vi "数据查询_数据查询.vi"() -> ()   [LabVIEW 2016]
uses:
  <vilib>/Utility/miscctls.llb/LVPointTypeDef.ctl
  <vilib>/Utility/miscctls.llb/LVRowAndColumnUnsignedTypeDef.ctl
  <vilib>/addons/database/_DB Variant To Data/Database Variant To Data.xnode
panel:
  in  "工作模式":string(combo)="全部数据"
  out "连接的字符串":string
  out "选中数据表":string
  in  "查询":bool
  in  "结束日期":string="2020/01/01"
  in  "起始日期":string="2010/01/01"
  out "XY图":cluster{"data":timestamp[], "data":dbl[]}[](graph)
  in  "组合框":string(combo)
  out "数据表":string[][](table)
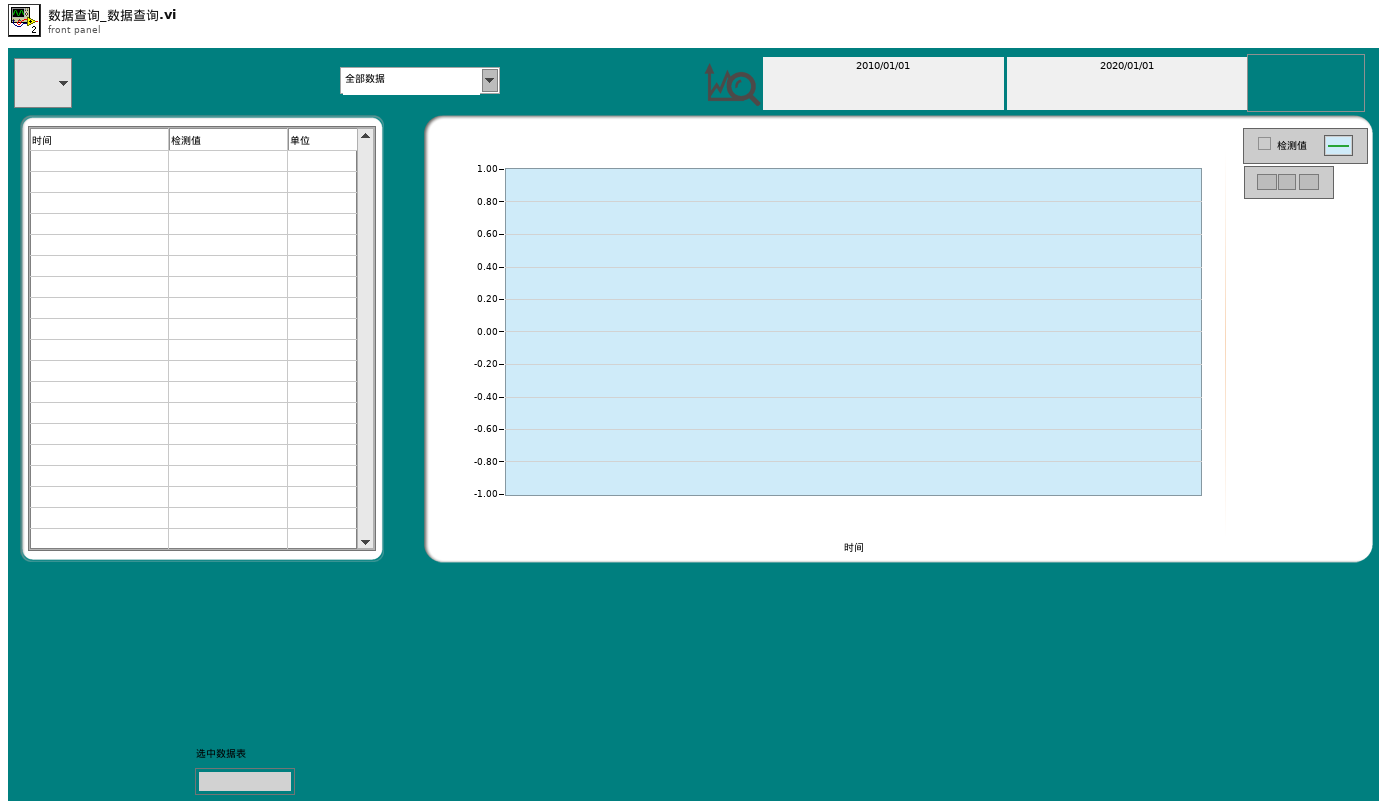
[diagram p1: front panel]
types:
  T1 = typedef "LVPointTypeDef.ctl" = cluster{"Horizontal":i16, "Vertical":i16}
  T2 = typedef "LVRowAndColumnUnsignedTypeDef.ctl" = cluster{"Row":u32, "Column":u32}
  T3 = typedef "LVPoint32TypeDef.ctl" = cluster{"Horizontal":i32, "Vertical":i32}
  T4 = typedef "LVPointDoubleTypeDef.ctl" = cluster{"Cursor X":dbl, "Cursor Y":dbl}
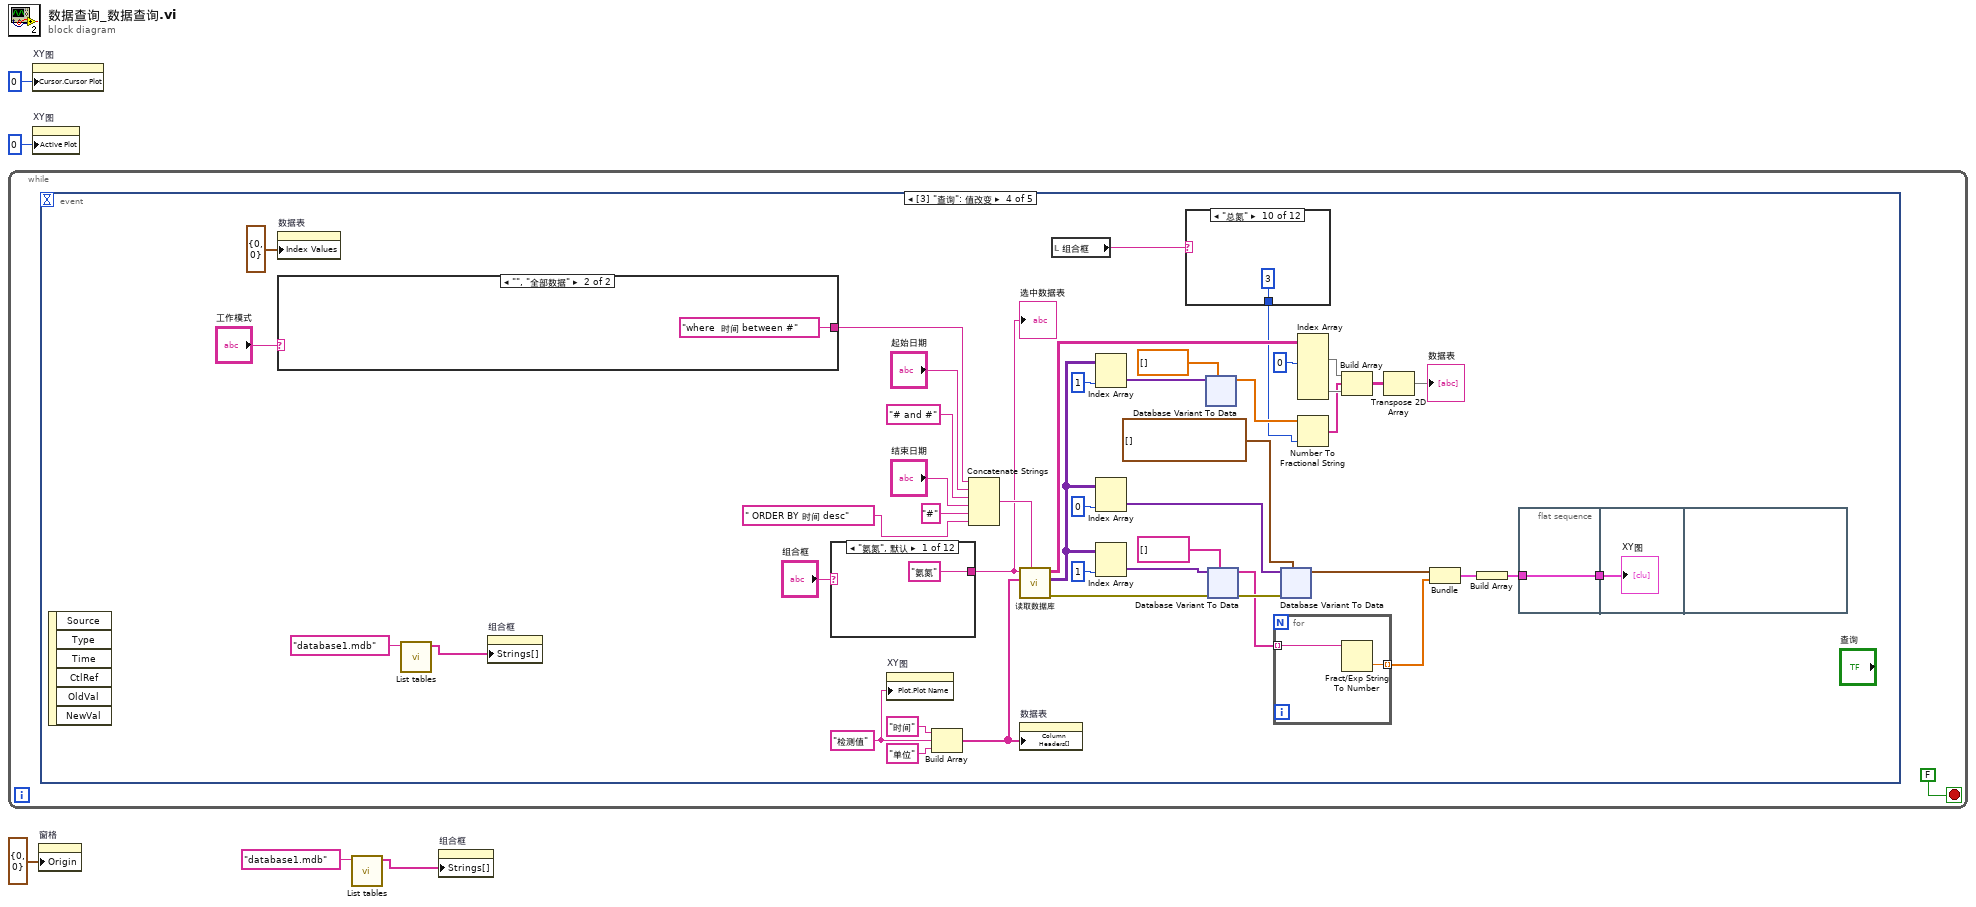
[diagram p0: block diagram]
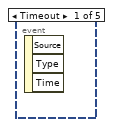
[diagram p2: hidden frame]
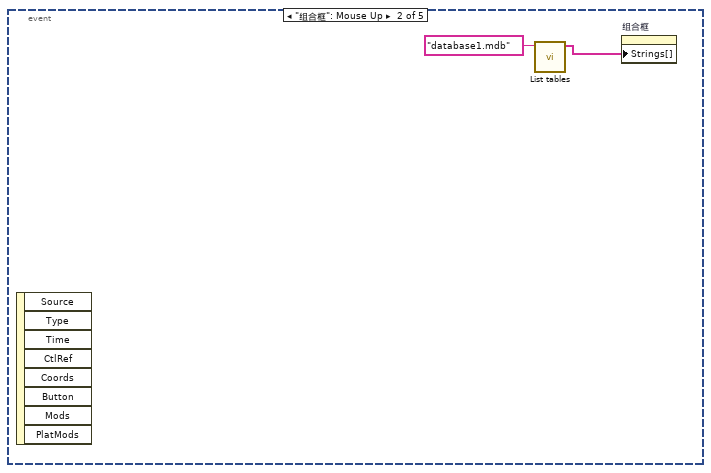
[diagram p3: hidden frame]
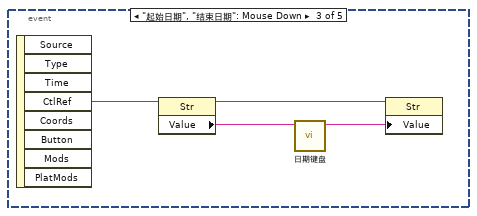
[diagram p4: hidden frame]
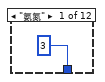
[diagram p5: hidden frame]
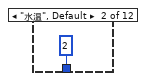
[diagram p6: hidden frame]
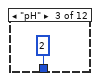
[diagram p7: hidden frame]
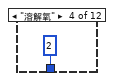
[diagram p8: hidden frame]
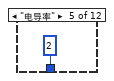
[diagram p9: hidden frame]
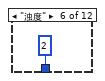
[diagram p10: hidden frame]
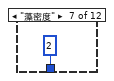
[diagram p11: hidden frame]
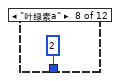
[diagram p12: hidden frame]
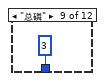
[diagram p13: hidden frame]
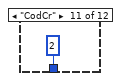
[diagram p14: hidden frame]
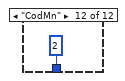
[diagram p15: hidden frame]
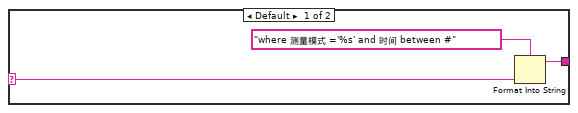
[diagram p16: hidden frame]
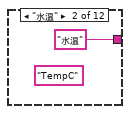
[diagram p17: hidden frame]
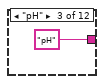
[diagram p18: hidden frame]
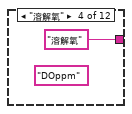
[diagram p19: hidden frame]
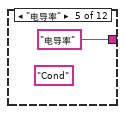
[diagram p20: hidden frame]
diagram:
  n1 = while {
    stop <- FALSE stop-if-true
    n2 = event shown="[3] \"查询\": 值改变" {
      selector: _ -> [_ _ _ _ _]
      dyn-events: _ -> [_ _ _ _ _]
      timeout: _ -> [_ _ _ _ _]
      event Timeout {
        n3 = event-data() -> ()  [unwired: 1 in, 3 out]
      }
      event "组合框": Mouse Up {
        n4 = event-data() -> ()  [unwired: 1 in, 8 out]
        n5 = call "List tables.vi"("database"="database1.mdb") -> ("tables"=w8:string[])  [unwired: 9 in, 1 out]
        n6 = property on="组合框" class="CmbBox"("Strings[]"=w8) -> ()  [unwired: 2 in, 2 out]
      }
      event "起始日期", "结束日期": Mouse Down {
        n7 = event-data() -> ("CtlRef"=w12:refnum<vi>)  [unwired: 1 in, 7 out]
        n8 = property class="Str"(reference=w12) -> (reference out=w10:refnum<vi>, "Value"=w11:string)  [unwired: 1 in, 1 out]
        n9 = call "日期键盘.vi"("原值"=w11) -> ("x+y"=w9:string)  [unwired: 10 in]
        n10 = property class="Str"(reference=w10, "Value"=w9) -> ()  [unwired: 1 in, 2 out]
      }
      event "查询": Value Change {
        w29 = "检测值"
        n11 = event-data() -> ()  [unwired: 1 in, 6 out]
        n12 = property on="数据表" class="Tbl (严格)"("Index Values"=T2 {"Row"=0, "Column"=0} ("索引值")) -> ()  [unwired: 2 in, 2 out]
        n13 = case shown="\"\", \"全部数据\"" "工作模式" {
          selector: "工作模式" -> [w72 _]
          tunnel: [w70 "where  时间 between #" ("condition")] -> w18
          frame Default {
            n14 = Format Into String(format string="where 测量模式 ='%s' and 时间 between #" ("condition"), w72) -> (resulting string=w70:string)  [unwired: 2 in, 1 out]
          }
          frame "", "全部数据" {
          }
        }
        n15 = call "List tables.vi"("database"="database1.mdb") -> ("tables"=w14:string[])  [unwired: 9 in, 1 out]
        n16 = property on="组合框" class="CmbBox"("Strings[]"=w14) -> ()  [unwired: 2 in, 2 out]
        n17 = case shown="\"氨氮\", 默认" "组合框" {
          tunnel: ["氨氮" "水温" "pH" "溶解氧" "电导率" "浊度" "藻密度" "叶绿素a" "总磷" "总氮" "CodCr" "CodMn"] -> w31
          frame "氨氮", Default {
          }
          frame "水温" {
            (unwired) "TempC"
          }
          frame "pH" {
          }
          frame "溶解氧" {
            (unwired) "DOppm"
          }
          frame "电导率" {
            (unwired) "Cond"
          }
          frame "浊度" {
            (unwired) "Turb"
          }
          frame "藻密度" {
            (unwired) "Algal"
          }
          frame "叶绿素a" {
            (unwired) "Chlor"
          }
          frame "总磷" {
            (unwired) "测量值"
          }
          frame "总氮" {
            (unwired) "测量值"
          }
          frame "CodCr" {
          }
          frame "CodMn" {
          }
        }
        "选中数据表" <- w31
        n18 = property on="XY图" class="XYGraph (严格)"("Plot.Plot Name"=w29) -> ()  [unwired: 2 in, 2 out]
        n19 = Build Array("时间", w29, "单位" ("元素")) -> (w32:string[])
        n20 = Concatenate Strings(w18, "起始日期", "# and #" ("condition"), "结束日期", "#" ("condition"), " ORDER BY 时间 desc" ("字符串")) -> (w56:string)
        n21 = call "读取数据库.vi"("condition"=w56, "显示项"=w32, "组合框"=w31) -> ("error out"=w47:errorcluster, "data"=w26:variant[][], "表格"=w39:string[][])  [unwired: 5 in, 1 out]
        n22 = property on="数据表" class="Tbl (严格)"("Column Headers[]"=w32) -> ()  [unwired: 2 in, 2 out]
        n23 = local read "组合框"() -> (w16:string)
        n24 = Index Array(array=w26, index (col)=1 ("禁用的索引 (列)")) -> (element=w24:variant[])  [unwired: 1 in]
        n25 = Index Array(array=w26, index (col)=0 ("禁用的索引 (列)")) -> (element=w50:variant[])  [unwired: 1 in]
        n26 = Index Array(array=w26, index (col)=1 ("禁用的索引 (列)")) -> (element=w48:variant[])  [unwired: 1 in]
        n27 = case shown="\"总氮\"" w16 {
          tunnel: [i16 3 ("精度(6)") i16 2 ("精度(6)") i16 2 ("精度(6)") i16 2 ("精度(6)") i16 2 ("精度(6)") i16 2 ("精度(6)") i16 2 ("精度(6)") i16 2 ("精度(6)") i16 3 ("精度(6)") i16 3 ("精度(6)") i16 2 ("精度(6)") i16 2 ("精度(6)")] -> w15
          frame "氨氮" {
          }
          frame "水温", Default {
          }
          frame "pH" {
          }
          frame "溶解氧" {
          }
          frame "电导率" {
          }
          frame "浊度" {
          }
          frame "藻密度" {
          }
          frame "叶绿素a" {
          }
          frame "总磷" {
          }
          frame "总氮" {
          }
          frame "CodCr" {
          }
          frame "CodMn" {
          }
        }
        n28 = xnode "Database Variant To Data"("database variant"=w24, "type"=sgl[] []) -> ("data"=w22:sgl[])  [unwired: 1 in, 1 out]
        n29 = xnode "Database Variant To Data"("database variant"=w48, "error in (no error)"=w47, "type"=string[] []) -> ("data"=w30:string[], "error out"=w46:errorcluster)
        n30 = for {
          tunnel: w30 -> [w113] mode=indexing
          tunnel: [w112] -> w17 mode=indexing
          n31 = Fract/Exp String To Number(string=w113) -> (number=w112:dbl)  [unwired: 3 in, 1 out]
        }
        n32 = xnode "Database Variant To Data"("database variant"=w50, "error in (no error)"=w46, "type"=timestamp[] []) -> ("data"=w41:timestamp[])  [unwired: 1 out]
        n33 = Index Array(array=w39, index (col) #1=0 ("禁用的索引 (列)")) -> (element #1=w37:string[], element #3=w27:string[])  [unwired: 5 in, 1 out]
        n34 = Number To Fractional String(number=w22, precision (6)=w15) -> (F-format string=w21:string[])  [unwired: 2 in]
        n35 = Build Array(w37, w21, w27) -> (w36:string[][])
        n36 = Transpose 2D Array(2D array=w36) -> (transposed array=→"数据表":string[][])
        n37 = Bundle("data"=w41, w17) -> (w42:cluster{"data":timestamp[], dbl[]})  [unwired: 1 in]
        n38 = Build Array(w42) -> (w43:cluster{"data":timestamp[], dbl[]}[])
        n39 = flat-sequence {
          tunnel: [w126] -> w44
          tunnel: w43 -> [w126]
          tunnel: w44 -> [w127]
          frame #0 {
          }
          frame #1 {
            "XY图" <- w127
          }
          frame #2 {
          }
        }
      }
      event "XY图": Mouse Move {
        w221 = "   " ("字符串")
        n40 = event-data() -> ("CtlRef"=w231:refnum<vi>, "Coords"=w230:T3)  [unwired: 1 in, 3 out]
        n41 = invoke class="XYGraph (严格)" method="Map Coords To XY"(reference=w231, "Coords"=w230) -> (reference out=w229:refnum<vi>, error out=w226:errorcluster, "XY"=w228:cluster{"X":dbl, "Y":dbl})  [unwired: 5 in, 4 out]
        n42 = property class="XYGraph (严格)"(reference=w229, error in=w226, "Cursor.Cursor Position"=w228) -> (error out=w227:errorcluster)  [unwired: 1 out]
        n43 = property on="XY图" class="XYGraph (严格)"(error in=w227) -> ("Cursor.Cursor Position"=w224:T4)  [unwired: 1 in, 2 out]
        n44 = Unbundle(w224) -> ("Cursor X"=w223:dbl, "Cursor Y"=w220:dbl)
        n45 = property on="XY图" class="XYGraph (严格)"() -> ("Plot.Plot Name"=w218:string)  [unwired: 2 in, 2 out]
        n46 = Format Date/Time String(seconds (now)=w223) -> (date/time string=w222:string)  [unwired: 2 in]
        n47 = Number To Fractional String(number=w220) -> (F-format string=w219:string)  [unwired: 3 in]
        n48 = Concatenate Strings(w218, w221, w222, w221, w219) -> (→"连接的字符串":string)
      }
    }
  }
  n49 = property on="XY图" class="XYGraph (严格)"("Cursor.Cursor Plot"=0 ("游标.游标关联曲线")) -> ()  [unwired: 2 in, 2 out]
  n50 = property on="XY图" class="XYGraph (严格)"("Active Plot"=u32 0 ("活动曲线")) -> ()  [unwired: 2 in, 2 out]
  n51 = property on="窗格" class="Pane"("Origin"=T1 {"Horizontal"=0, "Vertical"=0} ("原点")) -> ()  [unwired: 2 in, 2 out]
  n52 = call "List tables.vi"("database"="database1.mdb") -> ("tables"=w1:string[])  [unwired: 9 in, 1 out]
  n53 = property on="组合框" class="CmbBox"("Strings[]"=w1) -> ()  [unwired: 2 in, 2 out]
